vi "Ramp.vi"(6 "# of Samples":dbl=201.0 format="%#_13g", 9 "Start":dbl, 10 "Stop":dbl) -> (2 "Output":dbl[](array[numeric]))   [LabVIEW 2018]
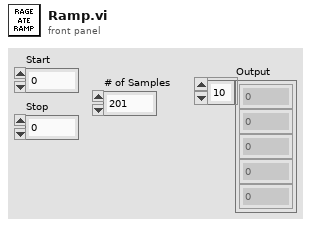
[diagram p1: front panel]
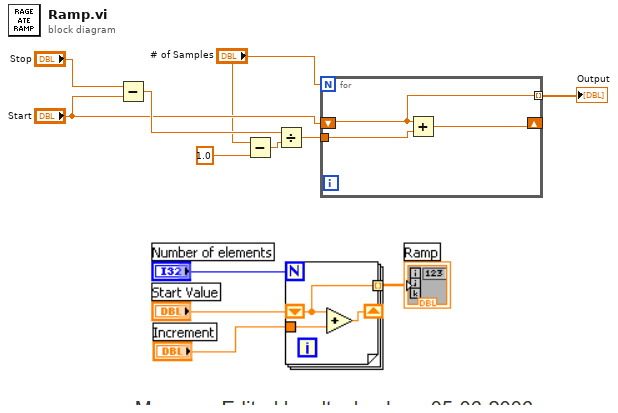
[diagram p0: block diagram]
diagram:
  n1 = Subtract(x="Stop", y="Start") -> (x-y=w6:dbl)
  n2 = Subtract(x="# of Samples", y=1.0 ("Points")) -> (x-y=w3:dbl)
  n3 = Divide(x=w6, y=w3) -> (x/y=w5:dbl)
  n4 = for {
    N: "# of Samples" -> [_]
    shift-right: [w10] -> _
    shift-left: "Start" -> [w11]
    tunnel: [w11] -> w8 mode=indexing
    tunnel: w5 -> [w9]
    n5 = Add(x=w11, y=w9) -> (x+y=w10:dbl)
  }
  "Output" <- w8
